vi "mouse_event.vi"() -> ()   [LabVIEW 2017]
uses:
  user32.dll
panel:
  in  "BARCODE STATION 3":string
  in  "Bool":bool
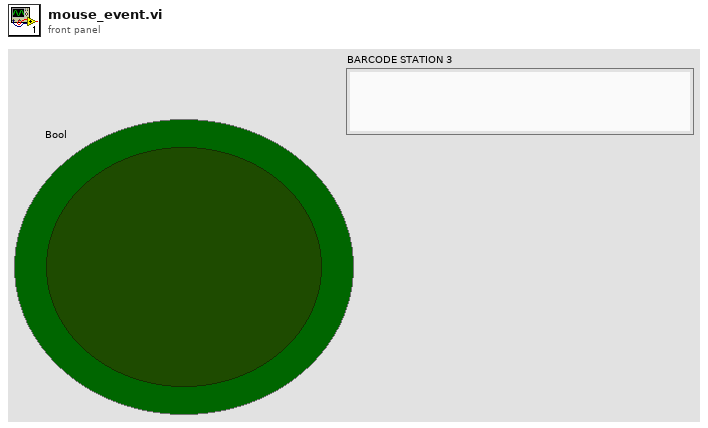
[diagram p1: front panel]
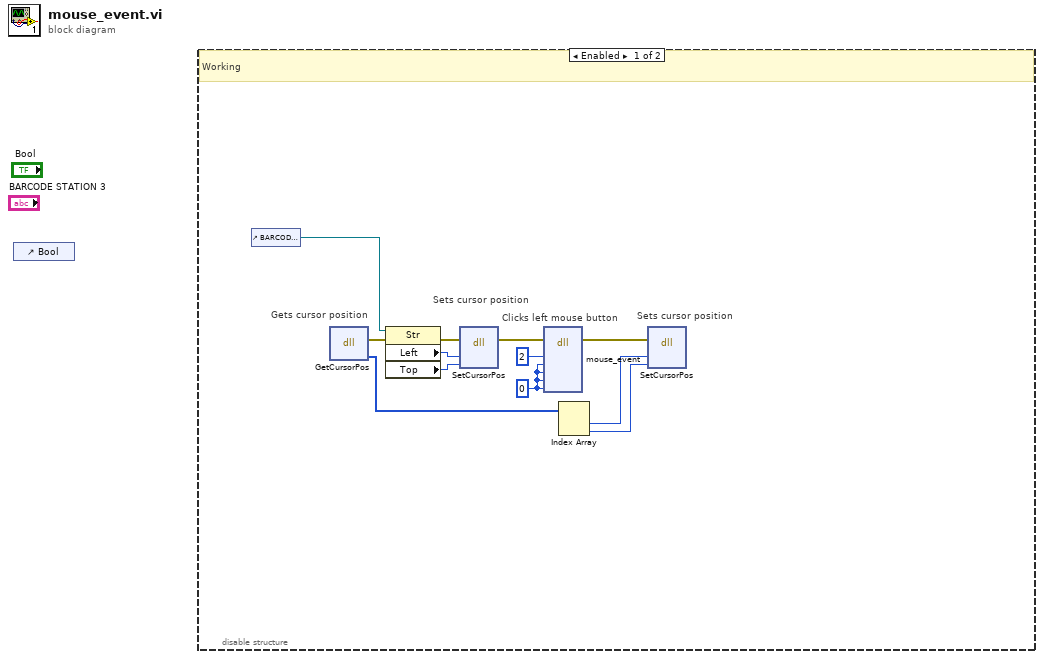
[diagram p0: block diagram]
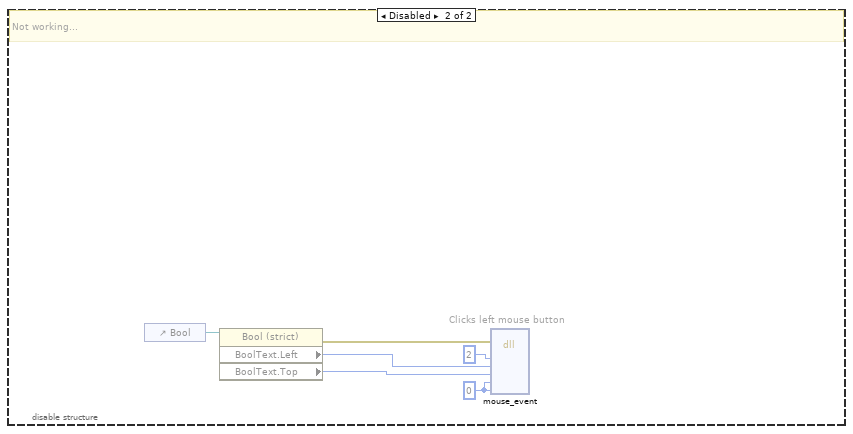
[diagram p2: hidden frame]
diagram:
  n1 = control-ref of="Bool"() -> ()  [unwired: 1 out]
  n2 = disable-structure shown="Enabled" {
    frame Enabled {
      w12 = u32 0 ("dy")
      # "Sets cursor position"
      # "Gets cursor position"
      # "Clicks left mouse button"
      # "Sets cursor position"
      # "Working"
      n3 = control-ref of="BARCODE STATION 3"() -> (w3:refnum<vi>)
      n4 = dll-call lib="User32.dll" fn="GetCursorPos" ("Move mouse to new pos")() -> (error out=w5:errorcluster, "POINT"=w8:i32[])  [unwired: 5 in, 1 out]
      n5 = property on="Property Node" class="Str"(reference=w3, error in=w5) -> (error out=w4:errorcluster, "Left"=w7:i32, "Top"=w6:i32)  [unwired: 1 out]
      n6 = dll-call lib="User32.dll" fn="SetCursorPos" ("Move mouse to new pos")(error in=w4, "dx"=w7, "dy"=w6) -> (error out=w9:errorcluster)  [unwired: 5 in, 1 out]
      n7 = dll-call lib="user32.dll" fn="mouse_event"(error in=w9, "dwFlags"=u32 2, "dx"=w12, "dy"=w12, "dwData"=w12, "dwExtraInfo"=w12) -> (error out=w11:errorcluster)  [unwired: 8 in, 1 out]
      n8 = Index Array(array=w8) -> (element #1=w1:i32, element #2=w2:i32)  [unwired: 2 in]
      n9 = dll-call lib="User32.dll" fn="SetCursorPos" ("Move mouse to new pos")(error in=w11, "dx"=w1, "dy"=w2) -> ()  [unwired: 5 in, 2 out]
    }
    frame Disabled {
      w16 = u32 0 ("dy")
      # "Clicks left mouse button"
      # "Not working..."
      n10 = control-ref of="Bool"() -> (w18:refnum<vi>)
      n11 = property on="Property Node" class="Bool (strict)"(reference=w18) -> (error out=w15:errorcluster, "BoolText.Left"=w14:i32, "BoolText.Top"=w13:i32)  [unwired: 1 in, 1 out]
      n12 = dll-call lib="user32.dll" fn="mouse_event"(error in=w15, "dwFlags"=u32 2, "dx"=w14, "dy"=w13, "dwData"=w16, "dwExtraInfo"=w16) -> ()  [unwired: 8 in, 2 out]
    }
  }
